vi "test Parsed XML to System Definition .vi"(8 "error in":errorcluster, 11 "TestCase in":refnum<class "Scripting.lvclass">) -> (0 "error out":errorcluster, 3 "TestCase out":refnum<class "Scripting.lvclass">)   [LabVIEW 2020, in "Scripting.lvclass"]
uses:
  Scripting.lvclass
  Shared/VS Channels Definition for All Labels on Hardware Channel.ctl
  Shared/VS Channels Definition for Label.ctl
  Shared/VS Channel Definition for Parameter.ctl
  Shared/Direction.ctl
  Shared/Parameter Definition.ctl
  Encoding and Decoding/Encoding.ctl
  Shared/Transfer Type.ctl
  Scripting.lvclass/Scripting.ctl
  <vilib>/addons/_JKI Toolkits/VI Tester/TestCase.llb/TestCase.lvclass
  Scripting/Ballard ARINC 429 Scripting.lvlib
  niveristand-custom-device-testing-tools/VeriStandTestUtilities/VeriStandTestUtilities.lvlib
  Encoding and Decoding/Encoding and Decoding.lvlib
  C:/Program Files (x86)/National Instruments/LabVIEW 2020/vi.lib/addons/_JKI Toolkits/VI Tester/TestCase.llb/TestCase.lvclass
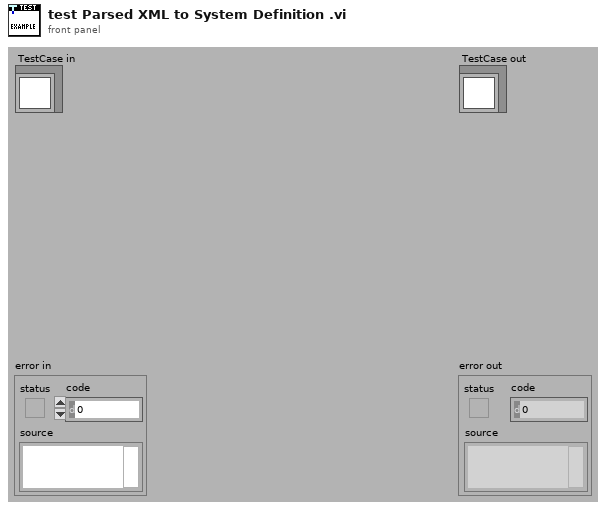
[diagram p1: front panel]
types:
  T1 = typedef "VS Channels Definition for All Labels on Hardware Channel.ctl" = cluster{"hardware channel":i32, "labels":T2[]}
  T2 = typedef "VS Channels Definition for Label.ctl" = cluster{"label (Dec)":i32, "parameters":T3[], "SDI value":u8, "SDI enabled":bool, "transfer type":T7}
  T3 = typedef "VS Channel Definition for Parameter.ctl" = cluster{"name":string, "direction":T4, "default value":dbl, "unit":string, "Parameter":T5}
  T4 = typedef "Direction.ctl" = enum16{"Rx", "Tx"}
  T5 = typedef "Parameter Definition.ctl" = cluster{"start index":i32, "size":i32, "encoding":T6, "signed":bool, "scale multiplier":dbl, "scale offset":dbl}
  T6 = typedef "Encoding and Decoding.lvlib/Encoding.ctl" = enum16{"BNR", "BCD", "Discrete"}
  T7 = typedef "Transfer Type.ctl" = enum16{"Scheduled", "Acyclic", "Block", "Strobe"}
  T8 = typedef "Custom Device API.lvlib/Custom Device Item Ref.ctl" = u64
  T9 = typedef "Label Properties.ctl" = cluster{"label (Dec)":i32, "SDI value":u8, "SDI enabled":bool}
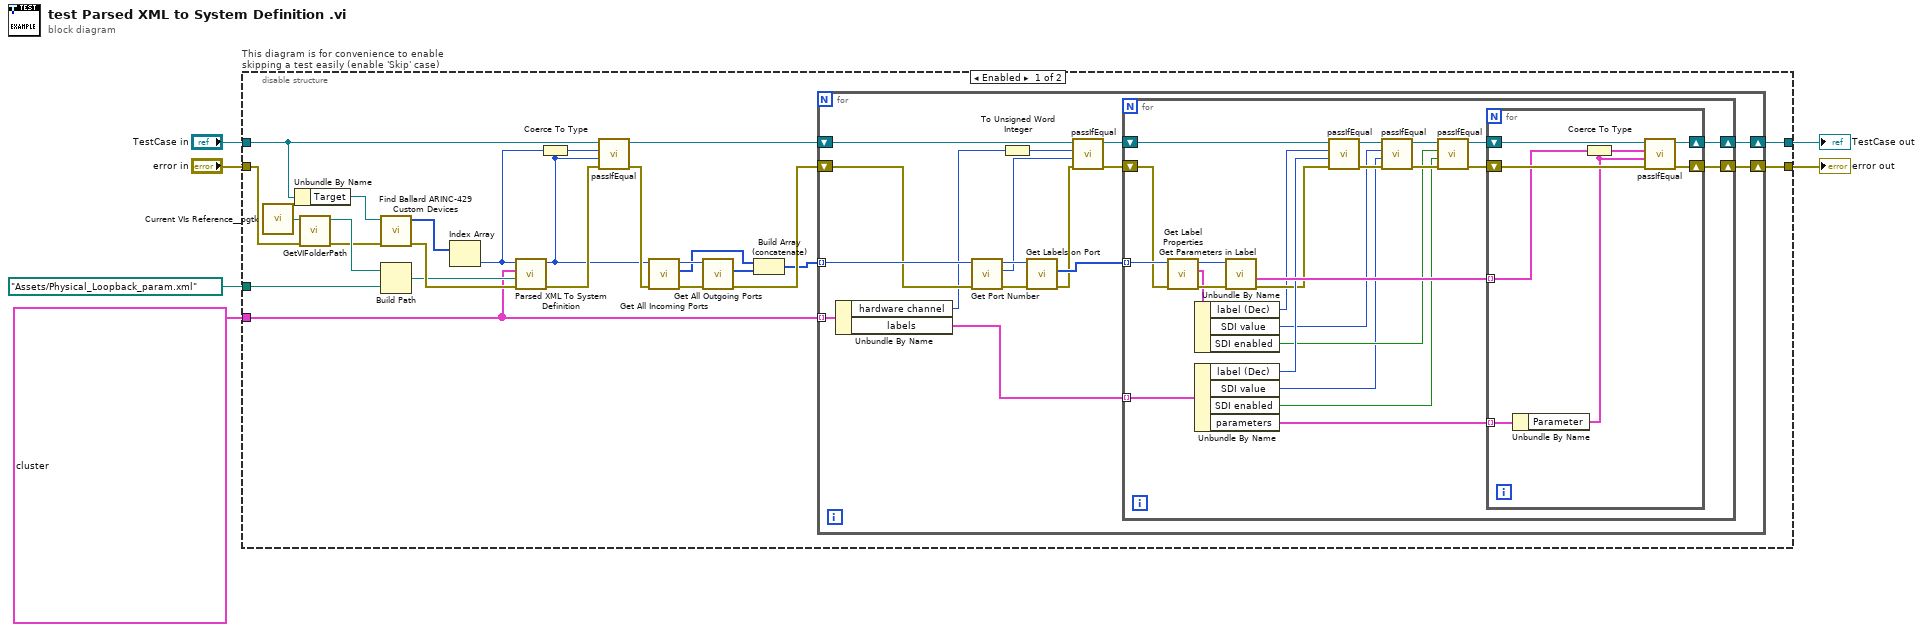
[diagram p0: block diagram]
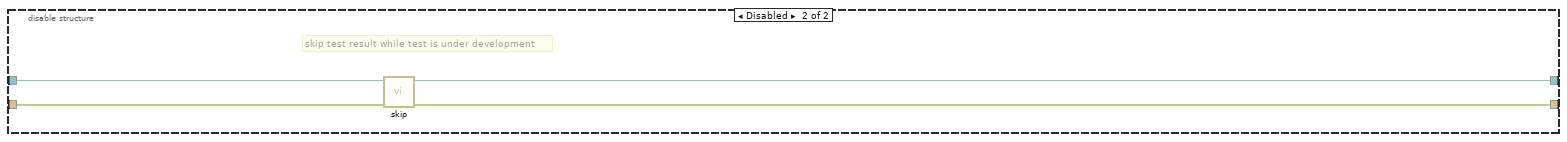
[diagram p2: hidden frame]
diagram:
  n1 = disable-structure "This diagram is for convenience to enable skipping a test easily (enable 'Skip' case)" shown="Enabled" {
    disable-tunnel: "TestCase in" -> [w22 w83]
    disable-tunnel: [w11 w81] -> w3
    disable-tunnel: [w9 w82] -> w5
    disable-tunnel: "error in" -> [w26 w80]
    disable-tunnel: T1[] [{"hardware channel"=0, "labels"=[{"label (Dec)"=134, "parameters"=[{"name"="Altitude_Rx", "direction"=enum."Rx", "default value"=0.0, "unit"="psi", "Parameter"={"start index"=18, "size"=10, "encoding"=enum."BNR", "signed"=TRUE, "scale multiplier"=16.0, "scale offset"=0.0}}, {"name"="SSM", "direction"=enum."Rx", "default value"=0.0, "unit"="", "Parameter"={"start index"=29, "size"=2, "encoding"=enum."BNR", "signed"=FALSE, "scale multiplier"=1.0, "scale offset"=0.0}}], "SDI value"=4, "SDI enabled"=FALSE, "transfer type"=enum."Scheduled"}]}, {"hardware channel"=2, "labels"=[{"label (Dec)"=135, "parameters"=[{"name"="Altitude_Rx", "direction"=enum."Rx", "default value"=0.0, "unit"="ft", "Parameter"={"start index"=10, "size"=19, "encoding"=enum."BCD", "signed"=TRUE, "scale multiplier"=1.0, "scale offset"=0.0}}, {"name"="SSM", "direction"=enum."Rx", "default value"=0.0, "unit"="", "Parameter"={"start index"=29, "size"=2, "encoding"=enum."BNR", "signed"=FALSE, "scale multiplier"=1.0, "scale offset"=0.0}}], "SDI value"=4, "SDI enabled"=FALSE, "transfer type"=enum."Scheduled"}]}, {"hardware channel"=4, "labels"=[{"label (Dec)"=136, "parameters"=[{"name"="Altitude_Rx", "direction"=enum."Rx", "default value"=0.0, "unit"="m", "Parameter"={"start index"=13, "size"=16, "encoding"=enum."BNR", "signed"=TRUE, "scale multiplier"=1.0, "scale offset"=0.0}}, {"name"="valid_Rx", "direction"=enum."Rx", "default value"=0.0, "unit"="", "Parameter"={"start index"=10, "size"=1, "encoding"=enum."Discrete", "signed"=FALSE, "scale multiplier"=1.0, "scale offset"=0.0}}, {"name"="current_Rx", "direction"=enum."Rx", "default value"=0.0, "unit"="", "Parameter"={"start index"=11, "size"=1, "encoding"=enum."Discrete", "signed"=FALSE, "scale multiplier"=1.0, "scale offset"=0.0}}, {"name"="SSM", "direction"=enum."Rx", "default value"=0.0, "unit"="", "Parameter"={"start index"=29, "size"=2, "encoding"=enum."BNR", "signed"=FALSE, "scale multiplier"=1.0, "scale offset"=0.0}}], "SDI value"=4, "SDI enabled"=FALSE, "transfer type"=enum."Scheduled"}]}, {"hardware channel"=17, "labels"=[{"label (Dec)"=134, "parameters"=[{"name"="Altitude_Tx", "direction"=enum."Tx", "default value"=0.0, "unit"="psi", "Parameter"={"start index"=18, "size"=10, "encoding"=enum."BNR", "signed"=TRUE, "scale multiplier"=16.0, "scale offset"=0.0}}], "SDI value"=4, "SDI enabled"=FALSE, "transfer type"=enum."Scheduled"}]}, {"hardware channel"=19, "labels"=[{"label (Dec)"=135, "parameters"=[{"name"="Altitude_Tx", "direction"=enum."Tx", "default value"=0.0, "unit"="ft", "Parameter"={"start index"=10, "size"=19, "encoding"=enum."BCD", "signed"=TRUE, "scale multiplier"=1.0, "scale offset"=0.0}}], "SDI value"=4, "SDI enabled"=FALSE, "transfer type"=enum."Scheduled"}]}, {"hardware channel"=21, "labels"=[{"label (Dec)"=136, "parameters"=[{"name"="Altitude_Tx", "direction"=enum."Tx", "default value"=0.0, "unit"="m", "Parameter"={"start index"=13, "size"=16, "encoding"=enum."BNR", "signed"=TRUE, "scale multiplier"=1.0, "scale offset"=0.0}}, {"name"="valid_Tx", "direction"=enum."Tx", "default value"=0.0, "unit"="", "Parameter"={"start index"=10, "size"=1, "encoding"=enum."Discrete", "signed"=FALSE, "scale multiplier"=1.0, "scale offset"=0.0}}, {"name"="current_Tx", "direction"=enum."Tx", "default value"=0.0, "unit"="", "Parameter"={"start index"=11, "size"=1, "encoding"=enum."Discrete", "signed"=FALSE, "scale multiplier"=1.0, "scale offset"=0.0}}], "SDI value"=4, "SDI enabled"=FALSE, "transfer type"=enum."Scheduled"}]}] ("ports") -> [w17 _]
    disable-tunnel: path "Assets/Physical_Loopback_param.xml" ("Absolute or Relative Path") -> [w24 _]
    frame Enabled {
      n2 = call <userlib>:"Current VIs Reference__ogtk.vi"() -> ("Current VI's reference"=w27:refnum<vi>)  [unwired: 5 in]
      n3 = Unbundle By Name(w22) -> ("Target"=w31:refnum<k24>)
      n4 = call "GetVIFolderPath.vi"("error in (no error)"=w26, "VI Reference in"=w27) -> ("error out"=w25:errorcluster, "VI Folder Path out"=w28:path)  [unwired: 8 in]
      n5 = call "Find Ballard ARINC-429 Custom Devices.vi"("error in"=w25, "target"=w31) -> ("error out"=w29:errorcluster, "Ballard ARINC-429 custom devices"=w30:u64[])  [unwired: 8 in]
      n6 = Build Path(base path=w28, name or relative path=w24) -> (appended path=w23:path)
      n7 = Index Array(array=w30) -> (element=w20:u64)  [unwired: 1 in]
      n8 = call "Parsed XML To System Definition.vi"("error in"=w29, "path to XML document"=w23, "ports"=w17, "custom device ref"=w20) -> ("error out"=w21:errorcluster, "custom device ref out"=w7:T8)  [unwired: 6 in]
      n9 = Coerce To Type(0:w20, 1:w7) -> (2:w8:T8)
      n10 = call-dynamic "passIfEqual.vi"("error in (no error)"=w21, "y"=w7, "x"=w8, "TestCase in"=w22) -> ("error out"=w19:errorcluster, "TestCase out"=w10:refnum<class "Scripting.lvclass">)  [unwired: 6 in]
      n11 = call "Get All Incoming Ports.vi"("error in"=w19, "Ballard ARINC 429 ref"=w7) -> ("error out"=w16:errorcluster, "Port refs"=w13:T8[], "Ballard ARINC 429 ref out"=w18:T8)  [unwired: 7 in]
      n12 = call "Get All Outgoing Ports.vi"("error in"=w16, "Ballard ARINC 429 ref"=w18) -> ("error out"=w15:errorcluster, "Port refs"=w14:T8[])  [unwired: 7 in, 1 out]
      n13 = Build Array (concatenate)(w13, w14) -> (w12:T8[])
      n14 = for {
        tunnel: w12 -> [w45] mode=indexing
        tunnel: w17 -> [w47] mode=indexing
        shift-right: [w42] -> w9
        shift-left: w15 -> [w44]
        shift-right: [w33] -> w11
        shift-left: w10 -> [w39]
        n15 = Unbundle By Name(w47) -> ("hardware channel"=w38:i32, "labels"=w40:T2[])
        n16 = call "Get Port Number.vi"("error in"=w44, "port ref in"=w45) -> ("error out"=w43:errorcluster, "port number"=w37:u16, "port ref out"=w46:T8)  [unwired: 6 in, 1 out]
        n17 = To Unsigned Word Integer(number=w38) -> (unsigned 16bit integer=w32:u16)
        n18 = call "Get Labels on Port.vi"("error in"=w43, "port ref"=w46) -> ("error out"=w36:errorcluster, "label references"=w41:T8[])  [unwired: 6 in, 2 out]
        n19 = call-dynamic "passIfEqual.vi"("error in (no error)"=w36, "y"=w37, "x"=w32, "TestCase in"=w39) -> ("error out"=w35:errorcluster, "TestCase out"=w34:refnum<class "Scripting.lvclass">)  [unwired: 6 in]
        n20 = for {
          shift-right: [w52] -> w42
          shift-left: w35 -> [w70]
          tunnel: w41 -> [w71] mode=indexing
          tunnel: w40 -> [w67] mode=indexing
          shift-right: [w53] -> w33
          shift-left: w34 -> [w59]
          n21 = call "Get Label Properties.vi"("error in"=w70, "label ref in"=w71) -> ("error out"=w69:errorcluster, "label properties"=w66:T9, "label ref out"=w68:T8)  [unwired: 7 in]
          n22 = Unbundle By Name(w66) -> ("label (Dec)"=w51:i32, "SDI value"=w56:u8, "SDI enabled"=w50:bool)
          n23 = Unbundle By Name(w67) -> ("label (Dec)"=w58:i32, "SDI value"=w48:u8, "SDI enabled"=w49:bool, "parameters"=w64:T3[])
          n24 = call "Get Parameters in Label.vi"("error in"=w69, "label ref"=w68) -> ("error out"=w57:errorcluster, "parameter definitions"=w65:T5[])  [unwired: 6 in, 2 out]
          n25 = call-dynamic "passIfEqual.vi"("error in (no error)"=w57, "y"=w58, "x"=w51, "TestCase in"=w59) -> ("error out"=w60:errorcluster, "TestCase out"=w61:refnum<class "Scripting.lvclass">)  [unwired: 6 in]
          n26 = call-dynamic "passIfEqual.vi"("error in (no error)"=w60, "y"=w48, "x"=w56, "TestCase in"=w61) -> ("error out"=w63:errorcluster, "TestCase out"=w62:refnum<class "Scripting.lvclass">)  [unwired: 6 in]
          n27 = call-dynamic "passIfEqual.vi"("error in (no error)"=w63, "y"=w49, "x"=w50, "TestCase in"=w62) -> ("error out"=w54:errorcluster, "TestCase out"=w55:refnum<class "Scripting.lvclass">)  [unwired: 6 in]
          n28 = for {
            tunnel: w65 -> [w76] mode=indexing
            tunnel: w64 -> [w79] mode=indexing
            shift-right: [w74] -> w53
            shift-left: w55 -> [w78]
            shift-right: [w75] -> w52
            shift-left: w54 -> [w77]
            n29 = Unbundle By Name(w79) -> ("Parameter"=w72:T5)
            n30 = Coerce To Type(0:w76, 1:w72) -> (2:w73:T5)
            n31 = call-dynamic "passIfEqual.vi"("error in (no error)"=w77, "y"=w72, "x"=w73, "TestCase in"=w78) -> ("error out"=w75:errorcluster, "TestCase out"=w74:refnum<class "Scripting.lvclass">)  [unwired: 6 in]
          }
        }
      }
    }
    frame Disabled {
      # "skip test result while test is under development"
      n32 = call <vilib>:"skip.vi"("error in (no error)"=w80, "TestCase in"=w83) -> ("error out"=w82:errorcluster, "TestCase out"=w81:refnum<class "Scripting.lvclass">)  [unwired: 8 in]
    }
  }
  "error out" <- w5
  "TestCase out" <- w3
